vi "SimClimb.vi"() -> ()   [LabVIEW 2023]
uses:
  <vilib>/Rock Robotics/WPI/ThirdParty/JAS_Junk/TrajLib/Enum/DCMOTOR_TYPES_ENUM.ctl
  <vilib>/Rock Robotics/WPI/ThirdParty/JAS_Junk/TrajLib/VI/Util_GetTime_U32.vi
  <vilib>/Rock Robotics/WPI/ThirdParty/JAS_Junk/TrajLib/SlewRateLimiter_New.vi
  <vilib>/Rock Robotics/WPI/ThirdParty/JAS_Junk/TrajLib/SlewRateLimiter_Reset.vi
  <vilib>/Rock Robotics/WPI/ThirdParty/JAS_Junk/TrajLib/SlewRateLimiter_Calculate.vi
  <vilib>/Rock Robotics/WPI/ThirdParty/JAS_Junk/TrajLib/SlewRateLimiter_SetRate.vi
  <vilib>/Rock Robotics/WPI/ThirdParty/JAS_Junk/TrajLib/VI/Util_GetTime_U64.vi
  <vilib>/Rock Robotics/WPI/ThirdParty/JAS_Junk/TrajLib/Trajectory_Library.lvlib
panel:
  out "Right Position\nInches (PV) 2":dbl format="%13.1f"
  out "Right Motor \nDmd (CO)":dbl format="%10.3f"
  in  "Top":bool
  in  "Bottom":bool
  in  "Down":bool
  in  "Up":bool
  out "R At Setpoint":bool
  out "R Rev / Lo Lim":bool
  out "R Fwd / Hi Lim":bool
  out "R Climb Control":T1(graph)
  out "Motor Current":dbl
  out "L Rev / Lo Lim":bool
  out "L Fwd / Hi Lim":bool
  out "Climb Demand (SP)\nInches":dbl
  out "Battery Voltage":dbl format="%10.1f"
  out "L Climb Control":T1(graph)
  out "Left Position\nInches (PV)":dbl format="%13.1f"
  out "L AtSetpoint":bool
  out "Left Motor \nDmd (CO)":dbl format="%10.3f"
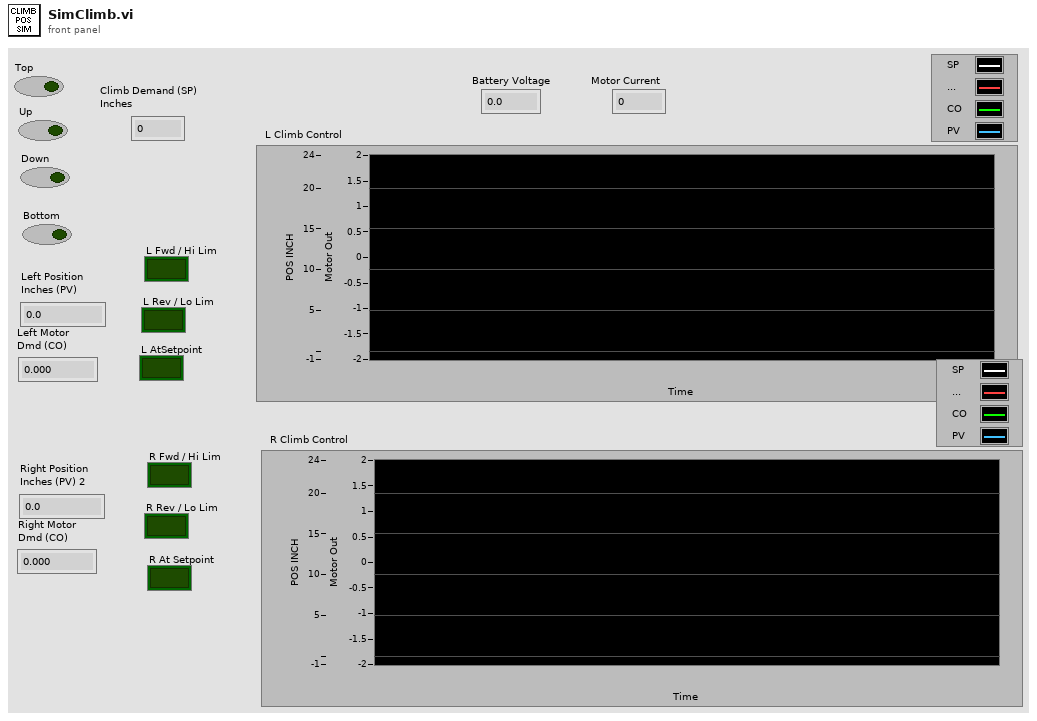
[diagram p1: front panel]
types:
  T1 = cluster{"Setpoint":dbl, "FeedForward":dbl, "CO-ControlOutput":dbl, "Velocity_RPM":dbl}
  T2 = cluster{"LeftSensorPosition":dbl, "RightSensorPosition":dbl, "LeftSensorVelocity":dbl, "RightSensorVelocity":dbl, "LeftRevLimit":bool, "LeftFwdLimit":bool, "RightRevLimit":bool, "RightFwdLimit":bool}
  T3 = typedef "Trajectory_Library.lvlib/DCMOTOR_TYPES_ENUM.ctl" = enum16{"CIM", "AndyMark 9015", "Andy Mark RS 775 125", "Bag", "BaneBots RS 550", "BaneBots RS 775", "Falcon 500", "Mini CIM", "NEO", "NEO 550", "Romi BuiltIn", "Vex 775 Pro", "Snow Blower AM 2235A", "Bosch Seat AM 3493"}
  T4 = typedef "Trajectory_Library.lvlib/LINEAR_SYSTEM_ID_ELEVATOR_MODEL.CTL" = cluster{"DCMOTOR_TYPES":T3, "Num Motors":i32, "WinchRadias_Meters":dbl, "mass_Kg":dbl, "Gearing":dbl}
  T5 = typedef "Trajectory_Library.lvlib/ELEVATOR_SIM_SIMULATION_PARAMS.ctl" = cluster{"MinHeight_Meters":dbl, "MaxHeight_Meters":dbl, "Measurment StdDev":dbl, "SimulateGravity":bool}
  T6 = cluster{"DesiredHeight":dbl, "LeftOnTarget":bool, "RightOnTarget":bool}
  T7 = cluster{"LeftMotorOutput":dbl, "RightMotorOutput":dbl}
  T8 = cluster{"DesiredHeight":dbl, dbl, "LeftMotorOutput":dbl, dbl}
  T9 = cluster{"DesiredHeight":dbl, dbl, "RightMotorOutput":dbl, dbl}
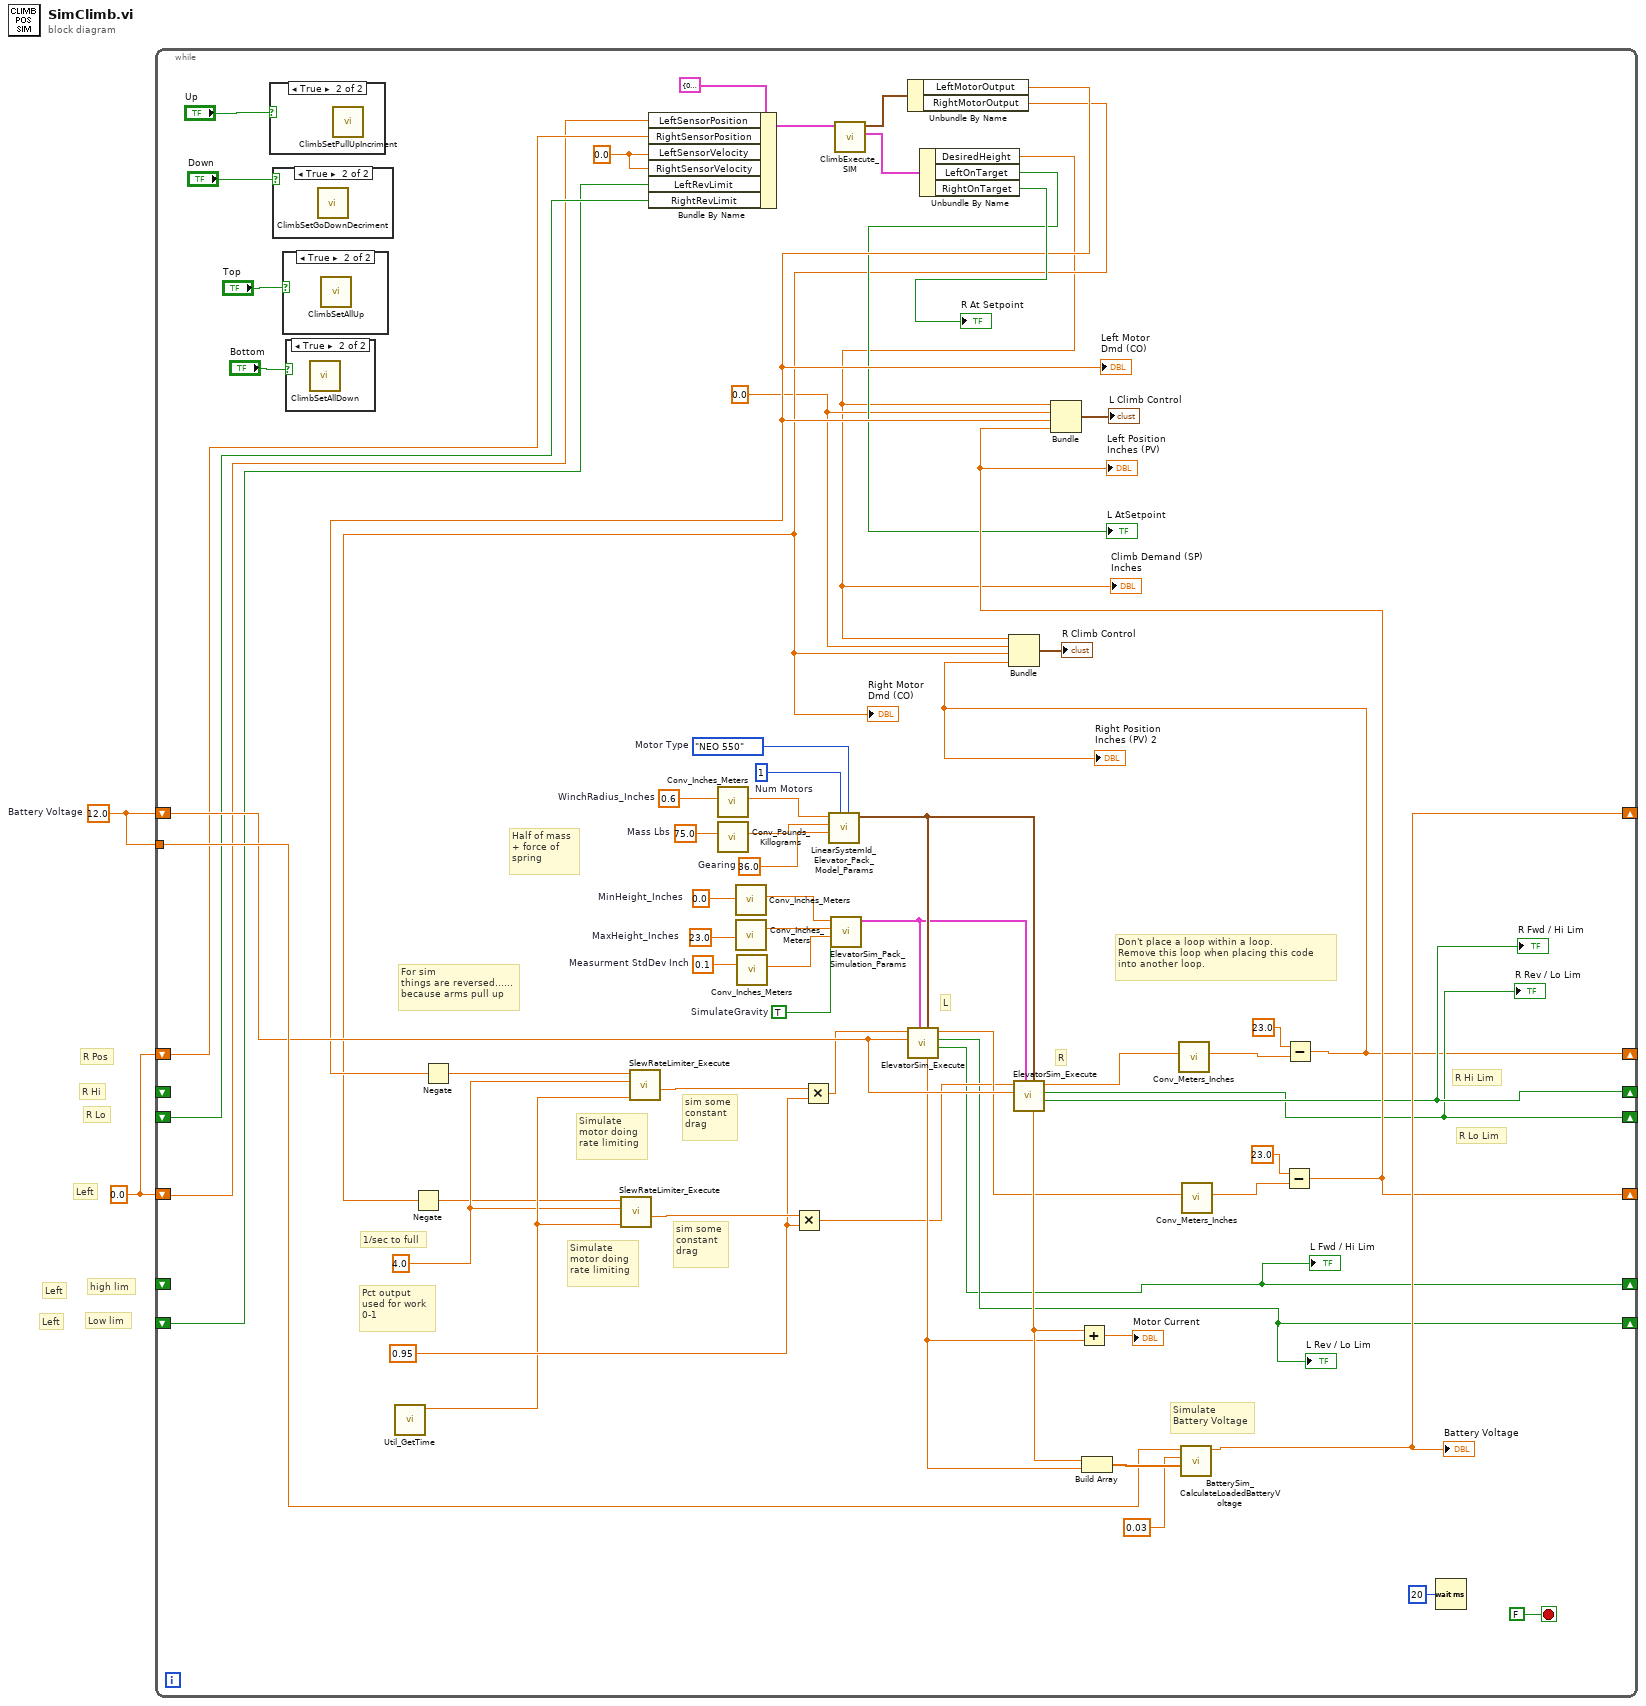
[diagram p0: block diagram]
diagram:
  w1 = 0.0 ("Degrees")
  w2 = 12.0  # Battery Voltage
  # "R Pos"
  # "R Lo"
  # "R Hi"
  # "Left"
  # "Left"
  # "Left"
  # "Low lim"
  # "high lim"
  n1 = while {
    shift-right: [w50] -> _
    shift-left: w2 -> [w47]
    shift-right: [w28] -> _
    shift-left: w1 -> [w9]
    tunnel: w2 -> [w49]
    shift-right: [w26] -> _
    shift-left: _ -> [_]
    shift-right: [w27] -> _
    shift-left: _ -> [w8]
    shift-right: [w6] -> _
    shift-left: w1 -> [w11]
    shift-right: [w24] -> _
    shift-left: _ -> [_]
    shift-right: [w23] -> _
    shift-left: _ -> [w10]
    stop <- FALSE stop-if-true
    w7 = 0.0 ("LeftSensorVelocity")
    w4 = 0.0
    w55 = 0.0  # MinHeight_Inches
    w56 = 23.0  # MaxHeight_Inches
    w57 = 0.1  # Measurment StdDev Inch
    w63 = TRUE  # SimulateGravity
    w61 = 0.6  # WinchRadius_Inches
    w64 = 36.0  # Gearing
    w59 = 75.0  # Mass Lbs
    w65 = 1  # Num Motors
    w66 = DCMOTOR_TYPES_ENUM."NEO 550"  # Motor Type
    w36 = 4.0 ("y")
    w38 = 0.95 ("y")
    # "For sim\nthings are reversed......\nbecause arms pull up"
    # "Simulate\nmotor doing\nrate limiting"
    # "sim some\nconstant\ndrag"
    # "R Lo Lim"
    # "R Hi Lim"
    # "R"
    # "L"
    # "Half of mass\n+ force of \nspring"
    # "Don't place a loop within a loop. \nRemove this loop when placing this code\ninto another loop."
    # "1/sec to full"
    # "Simulate\nBattery Voltage"
    # "Pct output\nused for work\n0-1"
    # "Simulate\nmotor doing\nrate limiting"
    # "sim some\nconstant\ndrag"
    n2 = case shown="True" "Up" {
      frame False {
      }
      frame True {
        n3 = call "ClimbSetPullUpIncriment.vi"() -> ()  [unwired: 11 in, 1 out]
      }
    }
    n4 = case shown="True" "Down" {
      frame False {
      }
      frame True {
        n5 = call "ClimbSetGoDownDecriment.vi"() -> ()  [unwired: 11 in, 1 out]
      }
    }
    n6 = case shown="True" "Top" {
      frame False {
      }
      frame True {
        n7 = call "ClimbSetAllUp.vi"() -> ()  [unwired: 11 in, 1 out]
      }
    }
    n8 = case shown="True" "Bottom" {
      frame False {
      }
      frame True {
        n9 = call "ClimbSetAllDown.vi"() -> ()  [unwired: 11 in, 1 out]
      }
    }
    n10 = call <vilib>:"Util_GetTime.vi"() -> ("FPGA_Time_Seconds"=w37:dbl)  [unwired: 9 in, 2 out]
    n11 = Bundle By Name(cluster=T2 {"LeftSensorPosition"=0.0, "RightSensorPosition"=0.0, "LeftSensorVelocity"=0.0, "RightSensorVelocity"=0.0, "LeftRevLimit"=FALSE, "LeftFwdLimit"=FALSE, "RightRevLimit"=FALSE, "RightFwdLimit"=FALSE} ("Inputs"), "LeftSensorPosition"=w9, "RightSensorPosition"=w11, "LeftSensorVelocity"=w7, "RightSensorVelocity"=w7, "LeftRevLimit"=w8, "RightRevLimit"=w10) -> (w12:T2)
    n12 = call <vilib>:"Conv_Inches_Meters.vi"("INCH"=w61) -> ("Meters"=w60:dbl)  [unwired: 10 in]
    n13 = call <vilib>:"Conv_Pounds_Killograms.vi"("Pounds"=w59) -> ("Killograms"=w58:dbl)  [unwired: 10 in]
    n14 = call <vilib>:"Conv_Inches_Meters.vi"("INCH"=w55) -> ("Meters"=w54:dbl)  [unwired: 10 in]
    n15 = call <vilib>:"Conv_Inches_Meters.vi"("INCH"=w56) -> ("Meters"=w53:dbl)  [unwired: 10 in]
    n16 = call <vilib>:"Conv_Inches_Meters.vi"("INCH"=w57) -> ("Meters"=w52:dbl)  [unwired: 10 in]
    n17 = call <vilib>:"LinearSystemId_Elevator_Pack_Model_Params.vi"("DCMOTOR_TYPES"=w66, "Num Motors"=w65, "Gearing"=w64, "mass_Kg"=w58, "WinchRadius_Meters"=w60) -> ("Elevator_Model _Params"=w62:T4)  [unwired: 6 in]
    n18 = call <vilib>:"ElevatorSim_Pack_Simulation_Params.vi"("SimulateGravity"=w63, "Measurment StdDev"=w52, "MaxHeight_Meters"=w53, "MinHeight_Meters"=w54) -> ("ElevatorSim_Simulation _Params"=w35:T5)  [unwired: 7 in]
    n19 = call "ClimbExecute_SIM.vi"("Inputs"=w12) -> ("InfoOutput"=w17:T6, "Outputs"=w18:T7)  [unwired: 8 in, 1 out]
    n20 = Unbundle By Name(w18) -> ("LeftMotorOutput"=w15:dbl, "RightMotorOutput"=w5:dbl)
    "Left Motor \nDmd (CO)" <- w15
    "Right Motor \nDmd (CO)" <- w5
    n21 = Negate(x=w5) -> (-x=w33:dbl)
    n22 = Negate(x=w15) -> (-x=w34:dbl)
    n23 = call <vilib>:"SlewRateLimiter_Execute.vi"("Time"=w37, "PositiveRate"=w36, "Input"=w33) -> ("Output"=w40:dbl)  [unwired: 7 in, 1 out]
    n24 = call <vilib>:"SlewRateLimiter_Execute.vi"("Time"=w37, "PositiveRate"=w36, "Input"=w34) -> ("Output"=w67:dbl)  [unwired: 7 in, 1 out]
    n25 = Multiply(x=w40, y=w38) -> (x*y=w39:dbl)
    n26 = Multiply(x=w67, y=w38) -> (x*y=w41:dbl)
    n27 = call <vilib>:"ElevatorSim_Execute.vi"("LinearSystemID_Elevator_Model _Params"=w62, "ElevatorSim_Simulation _Params"=w35, "Battery Volts"=w47, "Motor Dmd"=w41) -> ("AtLowLimit"=w26:bool, "At HIgh LImit"=w27:bool, "ElevatorHeight_Meters"=w43:dbl, "Motor Current"=w45:dbl)  [unwired: 2 in, 2 out]
    "L Fwd / Hi Lim" <- w26
    "L Rev / Lo Lim" <- w27
    n28 = Unbundle By Name(w17) -> ("DesiredHeight"=w3:dbl, "LeftOnTarget"=→"L AtSetpoint":bool, "RightOnTarget"=→"R At Setpoint":bool)
    "Climb Demand (SP)\nInches" <- w3
    n29 = call <vilib>:"ElevatorSim_Execute.vi"("LinearSystemID_Elevator_Model _Params"=w62, "ElevatorSim_Simulation _Params"=w35, "Battery Volts"=w47, "Motor Dmd"=w39) -> ("AtLowLimit"=w24:bool, "At HIgh LImit"=w23:bool, "ElevatorHeight_Meters"=w42:dbl, "Motor Current"=w46:dbl)  [unwired: 2 in, 2 out]
    "R Fwd / Hi Lim" <- w24
    "R Rev / Lo Lim" <- w23
    n30 = Add(x=w46, y=w45) -> (x+y=→"Motor Current":dbl)
    n31 = Build Array(w46, w45) -> (w51:dbl[])
    n32 = call <vilib>:"Conv_Meters_Inches.vi"("Meters"=w42) -> ("Inches"=w31:dbl)  [unwired: 10 in]
    n33 = call <vilib>:"BatterySim_CalculateLoadedBatteryVoltage.vi"("Currents"=w51, "Resistance_Ohms"=0.03, "NominalVoltage"=w49) -> ("Voltage"=w50:dbl)  [unwired: 8 in]
    "Battery Voltage" <- w50
    n34 = call <vilib>:"Conv_Meters_Inches.vi"("Meters"=w43) -> ("Inches"=w29:dbl)  [unwired: 10 in]
    n35 = Subtract(x=23.0, y=w29) -> (x-y=w28:dbl)
    "Left Position\nInches (PV)" <- w28
    n36 = Bundle("DesiredHeight"=w3, w4, "LeftMotorOutput"=w15, w28) -> (→"L Climb Control":T8)  [unwired: 1 in]
    n37 = Subtract(x=23.0, y=w31) -> (x-y=w6:dbl)
    "Right Position\nInches (PV) 2" <- w6
    n38 = Bundle("DesiredHeight"=w3, w4, "RightMotorOutput"=w5, w6) -> (→"R Climb Control":T9)  [unwired: 1 in]
    n39 = Wait (ms)(milliseconds to wait=u32 20) -> ()  [unwired: 1 out]
  }
